vi "Papaleta.vi"() -> ()   [LabVIEW 2016]
doc: "Interfaz en Labview que emula la operación de un cajero automático basado en máquinas de estados por eventos, las cuales reducen el procesamiento de datos en el microprocesador.\nEsta cajero cuenta con las operaciones de Retiro de efectivo, Pago de tarjeta de crédito, Compra de tiempo Aire, Estado de cuenta, Donativos, Depósitos a otras cuentas y Salir, ademas de un inicio por contraseña por asteriscos."
uses:
  Control_1Enum.ctl
panel:
  out "unsigned 8bit integer":u8
  out "Tab Control":T1(tab)
  out "Anuncios":u8(ring)
  in  "Boton_Aceptar_Contrasena":bool
  in  "Contrasena":string
  in  "Salir":bool
  out "Adeudo_Tarjeta":dbl
  out "Credito_Disponible":dbl
  in  "Estado de cuenta":bool
  in  "Depositos a otras cuentas":bool
  in  "Donativos":bool
  in  "Comprar Tiempo Aire":bool
  in  "Pagar Tarjeta":bool
  in  "Retirar Efectivo":bool
  in  "Regresar_1":bool
  in  "Retirar_Efectivo":bool
  in  "Cantidad a Retirar":dbl min=0.0 max=10000.0
  out "Adeudo_Tarjeta 2":dbl
  out "Credito_Disponible 2":dbl
  in  "Regresar_2":bool
  in  "Monto_a_Pagar":dbl min=0.0 max=10000.0
  in  "Pago_Tarjeta_Crédito":bool
  out "Adeudo_Tarjeta 3":dbl
  out "Credito_Disponible 3":dbl
  in  "Regresar_3":bool
  out "Adeudo_Tarjeta 4":dbl
  out "Credito_Disponible 4":dbl
  in  "Recargar_100":bool
  in  "Recargar_200":bool
  in  "Recargar_300":bool
  in  "Recargar_500":bool
  in  "Regresar_4":bool
  out "Adeudo_Tarjeta 5":dbl
  out "Credito_Disponible 5":dbl
  in  "Donar 100":bool
  in  "Donar 200":bool
  in  "Donar 300":bool
  in  "Donar 500":bool
  in  "Fundacion a Donar":string(combo)="World Vision Mexico"
  in  "Regresar_5":bool
  in  "Boton_P":bool
  out "Cantidad":string
  in  "Persona a depositar":string(combo)="Adrian Barba"
  out "Adeudo_Tarjeta 6":dbl
  out "Credito_Disponible 6":dbl
  in  "Aceptar":bool
  in  "Borrar":bool
  in  "Boton_9":bool
  in  "Limpiar":bool
  in  "Boton_6":bool
  in  "Boton_0":bool
  in  "Boton_3":bool
  in  "Boton_8":bool
  in  "Boton_7":bool
  in  "Boton_5":bool
  in  "Boton_4":bool
  in  "Boton_2":bool
  in  "Boton_1":bool
  in  "Regresar_6":bool
  out "Transacciones":string
  in  "Inserte su tarjeta":bool
  out "Led_Parpadeante":bool
  # "BANCO NACIONAL DE UPIITA"
  # "INGRESE SU CLAVE"
  # "Contraseña"
  # "Operaciones a Realizar"
  # "Crédito Disponible"
  # "Adeudo de la Tarjeta"
  # "Retirar Crédito"
  # "Crédito Disponible"
  # "Adeudo de la Tarjeta"
  # "Realizar Pago de la Tarjeta"
  # "Crédito Disponible"
  # "Adeudo de la Tarjeta"
  # "Recargar Tiempo Aire"
  # "Crédito Disponible"
  # "Adeudo de la Tarjeta"
  # "Donaciones a la Caridad"
  # "Crédito Disponible"
  # "Adeudo de la Tarjeta"
  # "Adeudo de la Tarjeta"
  # "Crédito Disponible"
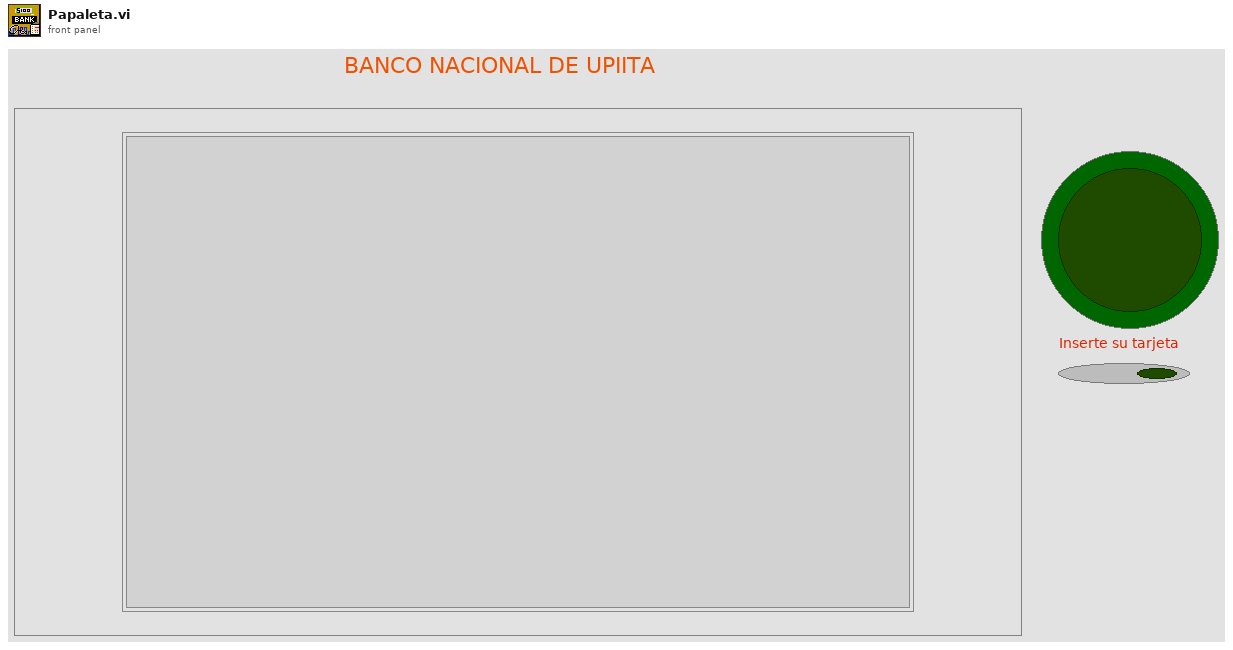
[diagram p1: front panel]
types:
  T1 = enum32{"Pant_Anuncios", "Pant_Contrasena", "Pant_Principal", "Pant_Retiro", "Pant_Pago", "Pant_Aire", "Pant_Donativos", "Pant_Depositos", "Pant_EdoCta"}
  T2 = typedef "Control_1Enum.ctl" = enum16{"Inicio", "Preguntar_Usuario", "Contrasena_valida", "Menu_Principal", "Menu_Retiro", "Menu_Pago", "Compra_TAire", "Donativos", "Depositos", "Estado_Cuenta"}
  T3 = cluster{"Credito Disponible":dbl, "Adeudo":dbl, "Primera Ejecucion":bool, "Transacciones":string, "Intentos":i8, "Pantalla":u8, "Cerrar Sesion":bool}
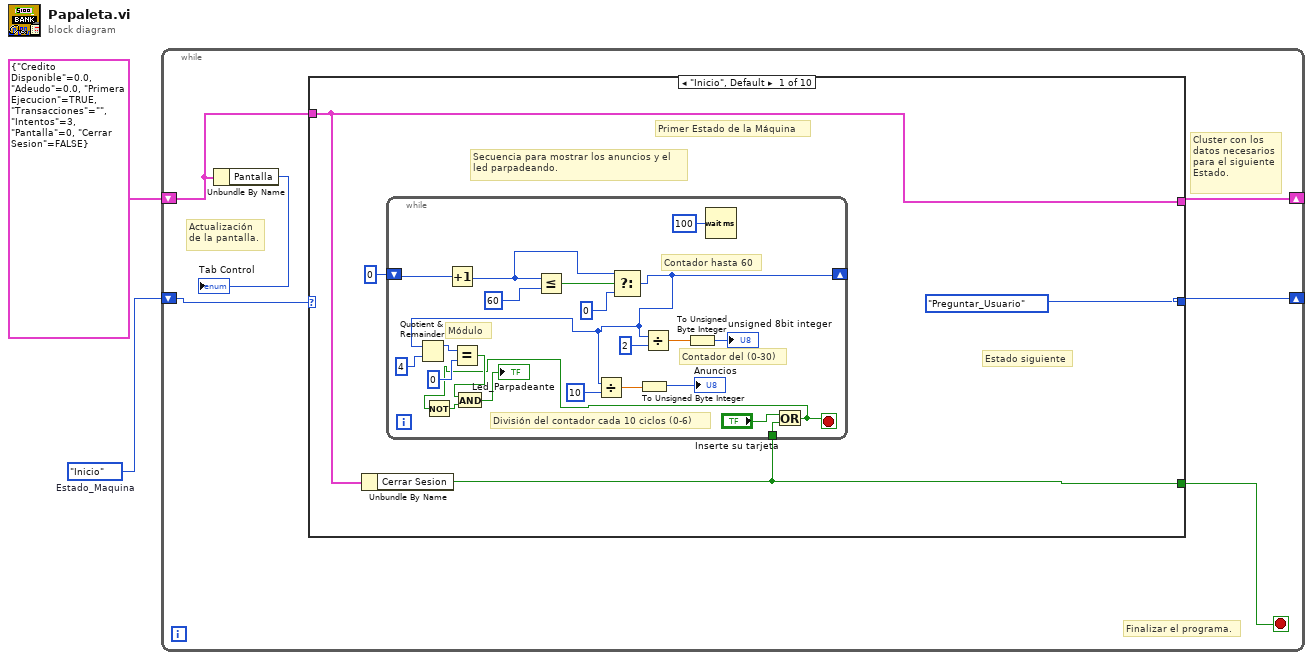
[diagram p0: block diagram]
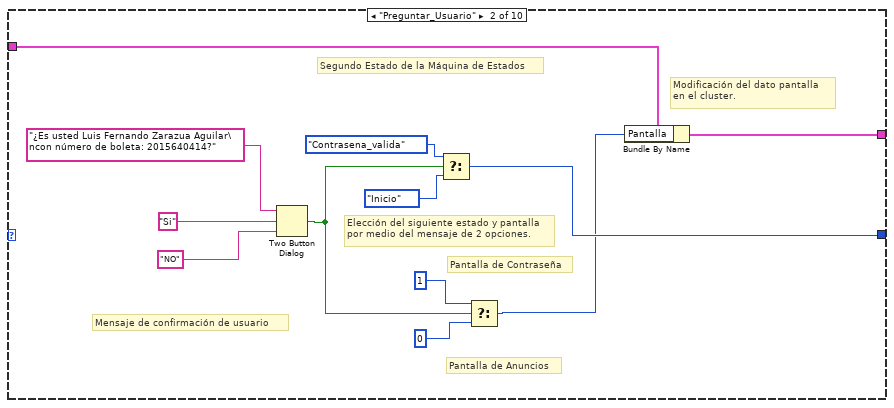
[diagram p2: hidden frame]
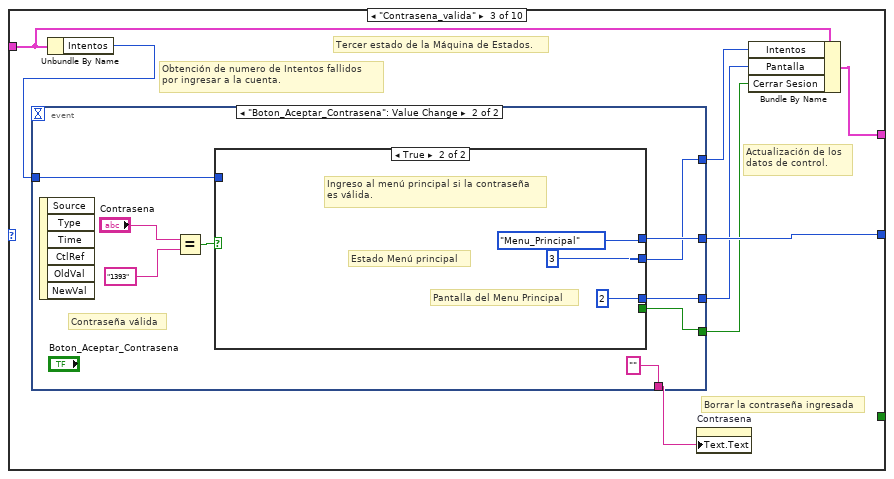
[diagram p3: hidden frame]
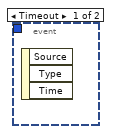
[diagram p4: hidden frame]
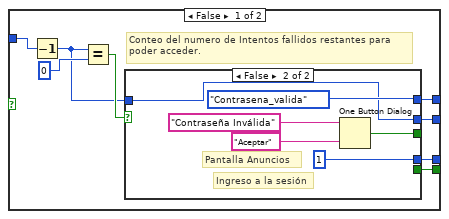
[diagram p5: hidden frame]
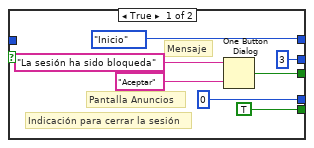
[diagram p6: hidden frame]
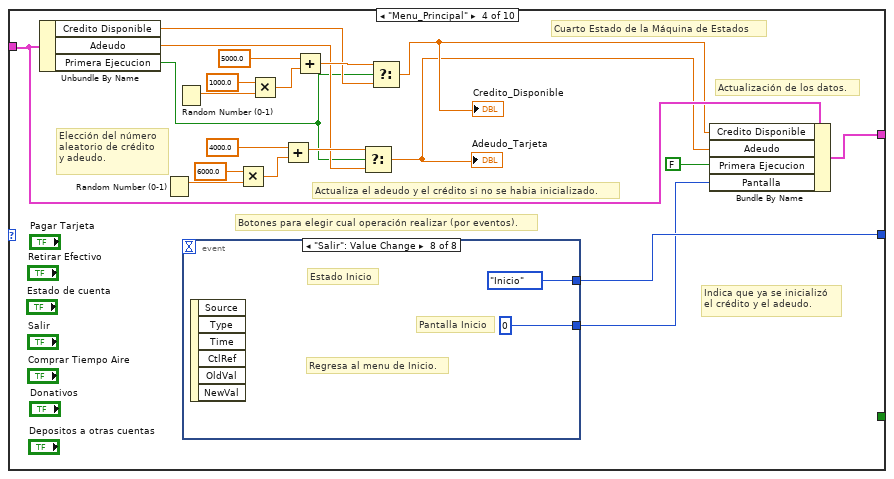
[diagram p7: hidden frame]
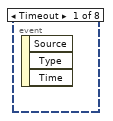
[diagram p8: hidden frame]
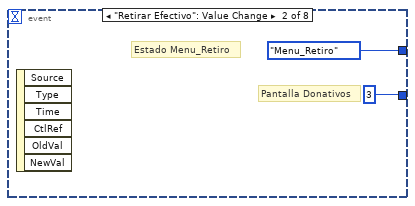
[diagram p9: hidden frame]
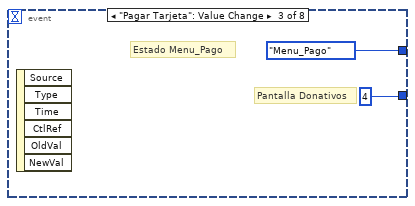
[diagram p10: hidden frame]
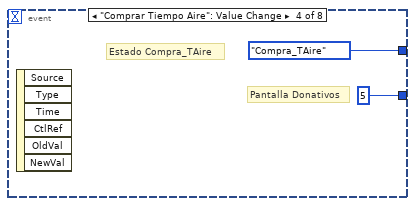
[diagram p11: hidden frame]
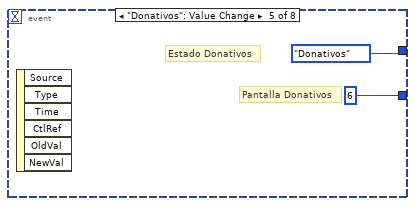
[diagram p12: hidden frame]
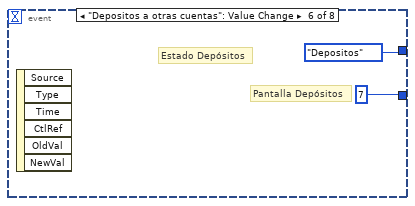
[diagram p13: hidden frame]
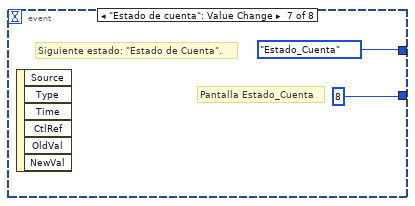
[diagram p14: hidden frame]
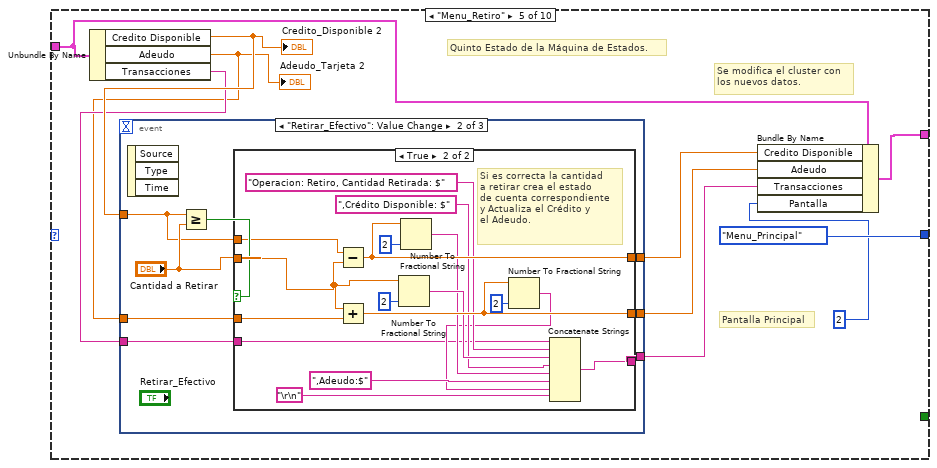
[diagram p15: hidden frame]
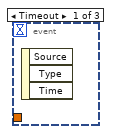
[diagram p16: hidden frame]
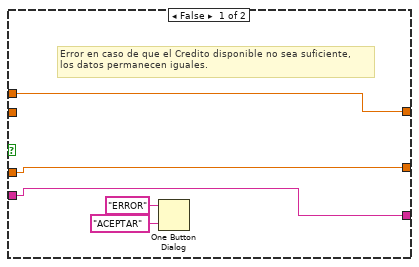
[diagram p17: hidden frame]
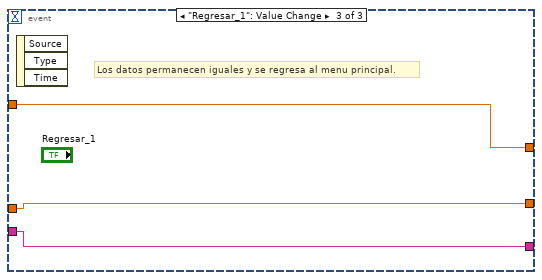
[diagram p18: hidden frame]
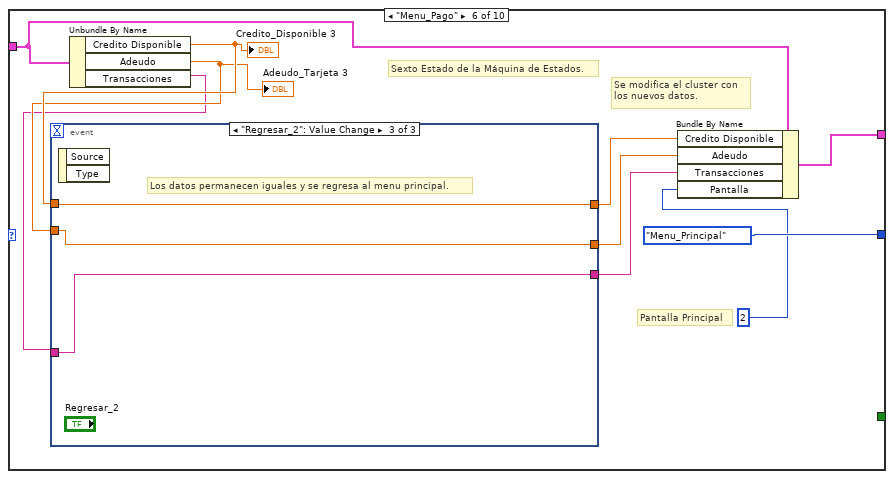
[diagram p19: hidden frame]
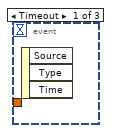
[diagram p20: hidden frame]
diagram:
  w2 = Control_1Enum."Inicio"  # Estado_Maquina
  n1 = while {
    shift-right: [w4] -> _
    shift-left: w2 -> [w3]
    shift-right: [w6] -> _
    shift-left: T3 {"Credito Disponible"=0.0, "Adeudo"=0.0, "Primera Ejecucion"=TRUE, "Transacciones"="", "Intentos"=3, "Pantalla"=0, "Cerrar Sesion"=FALSE} -> [w7]
    stop <- w5 stop-if-true
    # "Finalizar el programa."
    # "Cluster con los\ndatos necesarios\npara el siguiente\nEstado."
    # "Actualización \nde la pantalla."
    n2 = Unbundle By Name(w7) -> ("Pantalla"=→"Tab Control":u8)
    n3 = case shown="\"Inicio\", Default" w3 {
      tunnel: [Control_1Enum."Preguntar_Usuario" w40 w54 w97 Control_1Enum."Menu_Principal" Control_1Enum."Menu_Principal" Control_1Enum."Menu_Principal" Control_1Enum."Menu_Principal" w602 w774] -> w4
      tunnel: w7 -> [w10 w37 w51 w93 w123 w165 w211 w394 w584 w772]
      tunnel: [w10 w35 w49 w88 w122 w166 w210 w393 w583 w771] -> w6
      tunnel: [w9 _ _ _ _ _ _ _ _ _] -> w5
      frame "Inicio", Default {
        # "Secuencia para mostrar los anuncios y el\nled parpadeando."
        # "Estado siguiente"
        # "Primer Estado de la Máquina"
        n4 = Unbundle By Name(w10) -> ("Cerrar Sesion"=w9:bool)
        n5 = while {
          shift-right: [w22] -> _
          shift-left: i8 0 -> [w33]
          tunnel: w9 -> [w13]
          stop <- w15 stop-if-true
          # "Contador del (0-30)"
          # "Módulo"
          # "División del contador cada 10 ciclos (0-6)"
          # "Contador hasta 60"
          n6 = Increment(x=w33) -> (x+1=w30:i8)
          n7 = Less Or Equal?(x=w30, y=i8 60) -> (x <= y?=w31:bool)
          n8 = Select(t=w30, s=w31, f=i8 0) -> (s? t:f=w22:i8)
          n9 = Quotient & Remainder(x=w22, y=i8 4) -> (x-y*floor(x/y)=w20:i8)  [unwired: 1 out]
          n10 = Equal?(x=w20, y=i8 0) -> (x = y?=w17:bool)
          n11 = Divide(x=w22, y=i8 10) -> (x/y=w26:dbl)
          n12 = To Unsigned Byte Integer(number=w26) -> (unsigned 8bit integer=→"Anuncios":u8)
          n13 = Divide(x=w22, y=i8 2) -> (x/y=w24:dbl)
          n14 = To Unsigned Byte Integer(number=w24) -> (unsigned 8bit integer=→"unsigned 8bit integer":u8)
          n15 = Wait (ms)(milliseconds to wait=u32 100) -> ()  [unwired: 1 out]
          n16 = Or(x="Inserte su tarjeta", y=w13) -> (x .or. y?=w15:bool)
          n17 = Not(x=w15) -> (.not. x?=w16:bool)
          n18 = And(x=w17, y=w16) -> (x .and. y?=→"Led_Parpadeante":bool)
        }
      }
      frame "Preguntar_Usuario" {
        # "Modificación del dato pantalla\nen el cluster."
        # "Elección del siguiente estado y pantalla\npor medio del mensaje de 2 opciones."
        # "Mensaje de confirmación de usuario"
        # "Segundo Estado de la Máquina de Estados"
        # "Pantalla de Anuncios"
        # "Pantalla de Contraseña"
        n19 = Two Button Dialog(message="¿Es usted Luis Fernando Zarazua Aguilar\ncon número de boleta: 2015640414?", 1:"NO" ("F button name (\"Cancel\")"), 2:"Si" ("T button name (\"OK\")")) -> (T button?=w41:bool)
        n20 = Select(t=Control_1Enum."Contrasena_valida", s=w41, f=Control_1Enum."Inicio") -> (s? t:f=w40:T2)
        n21 = Select(t=u8 1, s=w41, f=0) -> (s? t:f=w36:i32)
        n22 = Bundle By Name(cluster=w37, "Pantalla"=w36) -> (w35:T3)
      }
      frame "Contrasena_valida" {
        # "Borrar la contraseña ingresada"
        # "Actualización de los\ndatos de control."
        # "Obtención de numero de Intentos fallidos\npor ingresar a la cuenta."
        # "Tercer estado de la Máquina de Estados."
        n23 = Unbundle By Name(w51) -> ("Intentos"=w52:i8)
        n24 = event shown="[1] \"Boton_Aceptar_Contrasena\": Value Change" {
          selector: _ -> [_ _]
          dyn-events: _ -> [_ _]
          timeout: _ -> [_ _]
          tunnel: [_ w60] -> w54
          tunnel: [_ w59] -> w48
          tunnel: [_ w58] -> w50
          tunnel: [_ "" ("Label.Text")] -> w53
          tunnel: [_ w56] -> w47
          tunnel: w52 -> [_ w55]
          event Timeout {
            n25 = event-data() -> ()  [unwired: 1 in, 3 out]
          }
          event "Boton_Aceptar_Contrasena": Value Change {
            # "Contraseña válida"
            n26 = event-data() -> ()  [unwired: 1 in, 6 out]
            n27 = Equal?(x="Contrasena", y="1393") -> (x = y?=w61:bool)
            n28 = case shown="True" w61 {
              tunnel: [w69 Control_1Enum."Menu_Principal"] -> w60
              tunnel: [w68 u8 2] -> w59
              tunnel: [w67 i8 3] -> w58
              tunnel: [w65 _] -> w56
              tunnel: w55 -> [w64 _]
              frame False {
                # "Conteo del numero de Intentos fallidos restantes para\npoder acceder."
                n29 = Decrement(x=w64) -> (x-1=w66:i8)
                n30 = Equal?(x=w66, y=i8 0) -> (x = y?=w70:bool)
                n31 = case shown="False" w70 {
                  tunnel: [Control_1Enum."Inicio" Control_1Enum."Contrasena_valida"] -> w69
                  tunnel: [u8 0 u8 1] -> w68
                  tunnel: [w74 w80] -> _
                  tunnel: [i8 3 w79] -> w67
                  tunnel: w66 -> [_ w79]
                  tunnel: [TRUE _] -> w65
                  frame True {
                    # "Mensaje"
                    # "Indicación para cerrar la sesión"
                    # "Pantalla Anuncios"
                    n32 = One Button Dialog(message="La sesión ha sido bloqueda", button name ("OK")="Aceptar") -> (true=w74:bool)
                  }
                  frame False {
                    # "Ingreso a la sesión"
                    # "Pantalla Anuncios"
                    n33 = One Button Dialog(message="Contraseña Inválida", button name ("OK")="Aceptar") -> (true=w80:bool)
                  }
                }
              }
              frame True {
                # "Estado Menú principal"
                # "Ingreso al menú principal si la contraseña\nes válida."
                # "Pantalla del Menu Principal"
              }
            }
          }
        }
        n34 = property on="Contrasena" class="Str"("Text.Text"=w53) -> ()  [unwired: 2 in, 2 out]
        n35 = Bundle By Name(cluster=w51, "Intentos"=w50, "Pantalla"=w48, "Cerrar Sesion"=w47) -> (w49:T3)
      }
      frame "Menu_Principal" {
        # "Actualización de los datos."
        # "Indica que ya se inicializó \nel crédito y el adeudo."
        # "Botones para elegir cual operación realizar (por eventos)."
        # "Actualiza el adeudo y el crédito si no se habia inicializado."
        # "Elección del número\naleatorio de crédito\ny adeudo."
        # "Cuarto Estado de la Máquina de Estados"
        n36 = Unbundle By Name(w93) -> ("Credito Disponible"=w96:dbl, "Adeudo"=w95:dbl, "Primera Ejecucion"=w94:bool)
        n37 = Random Number (0-1)() -> (number: 0 to 1=w103:dbl)
        n38 = Random Number (0-1)() -> (number: 0 to 1=w107:dbl)
        n39 = event shown="[7] \"Salir\": Value Change" {
          selector: _ -> [_ _ _ _ _ _ _ _]
          dyn-events: _ -> [_ _ _ _ _ _ _ _]
          timeout: _ -> [_ _ _ _ _ _ _ _]
          tunnel: [_ Control_1Enum."Menu_Retiro" Control_1Enum."Menu_Pago" Control_1Enum."Compra_TAire" Control_1Enum."Donativos" Control_1Enum."Depositos" Control_1Enum."Estado_Cuenta" Control_1Enum."Inicio"] -> w97
          tunnel: [_ u8 3 u8 4 u8 5 u8 6 u8 7 u8 8 u8 0] -> w89
          event Timeout {
            n40 = event-data() -> ()  [unwired: 1 in, 3 out]
          }
          event "Retirar Efectivo": Value Change {
            # "Estado Menu_Retiro"
            # "Pantalla Donativos"
            n41 = event-data() -> ()  [unwired: 1 in, 6 out]
          }
          event "Pagar Tarjeta": Value Change {
            # "Estado Menu_Pago"
            # "Pantalla Donativos"
            n42 = event-data() -> ()  [unwired: 1 in, 6 out]
          }
          event "Comprar Tiempo Aire": Value Change {
            # "Estado Compra_TAire"
            # "Pantalla Donativos"
            n43 = event-data() -> ()  [unwired: 1 in, 6 out]
          }
          event "Donativos": Value Change {
            # "Estado Donativos"
            # "Pantalla Donativos"
            n44 = event-data() -> ()  [unwired: 1 in, 6 out]
          }
          event "Depositos a otras cuentas": Value Change {
            # "Estado Depósitos"
            # "Pantalla Depósitos"
            n45 = event-data() -> ()  [unwired: 1 in, 6 out]
          }
          event "Estado de cuenta": Value Change {
            # "Siguiente estado: \"Estado de Cuenta\"."
            # "Pantalla Estado_Cuenta"
            n46 = event-data() -> ()  [unwired: 1 in, 6 out]
          }
          event "Salir": Value Change {
            # "Regresa al menu de Inicio."
            # "Estado Inicio"
            # "Pantalla Inicio"
            n47 = event-data() -> ()  [unwired: 1 in, 6 out]
          }
        }
        n48 = Multiply(x=6000.0, y=w103) -> (x*y=w100:dbl)
        n49 = Multiply(x=1000.0, y=w107) -> (x*y=w104:dbl)
        n50 = Add(x=4000.0, y=w100) -> (x+y=w98:dbl)
        n51 = Add(x=5000.0, y=w104) -> (x+y=w99:dbl)
        n52 = Select(t=w98, s=w94, f=w95) -> (s? t:f=w91:dbl)
        "Adeudo_Tarjeta" <- w91
        n53 = Select(t=w99, s=w94, f=w96) -> (s? t:f=w92:dbl)
        "Credito_Disponible" <- w92
        n54 = Bundle By Name(cluster=w93, "Credito Disponible"=w92, "Adeudo"=w91, "Primera Ejecucion"=FALSE, "Pantalla"=w89) -> (w88:T3)
      }
      frame "Menu_Retiro" {
        # "Se modifica el cluster con\nlos nuevos datos."
        # "Quinto Estado de la Máquina de Estados."
        # "Pantalla Principal"
        n55 = Unbundle By Name(w123) -> ("Credito Disponible"=w126:dbl, "Adeudo"=w124:dbl, "Transacciones"=w125:string)
        "Credito_Disponible 2" <- w126
        "Adeudo_Tarjeta 2" <- w124
        n56 = event shown="[1] \"Retirar_Efectivo\": Value Change" {
          selector: _ -> [_ _ _]
          dyn-events: _ -> [_ _ _]
          timeout: _ -> [_ _ _]
          tunnel: [_ w137 w164] -> w129
          tunnel: [_ w136 w163] -> w127
          tunnel: [_ w135 w162] -> w128
          tunnel: w126 -> [_ w132 w164]
          tunnel: w125 -> [_ w134 w162]
          tunnel: w124 -> [_ w133 w163]
          event Timeout {
            n57 = event-data() -> ()  [unwired: 1 in, 3 out]
          }
          event "Retirar_Efectivo": Value Change {
            n58 = event-data() -> ()  [unwired: 1 in, 3 out]
            n59 = Greater Or Equal?(x=w132, y="Cantidad a Retirar") -> (x >= y?=w138:bool)
            n60 = case shown="True" w138 {
              tunnel: "Cantidad a Retirar" -> [_ w155]
              tunnel: [w141 w159] -> w136
              tunnel: [w142 w158] -> w137
              tunnel: [w140 w161] -> w135
              tunnel: w134 -> [w140 w147]
              tunnel: w133 -> [w141 w146]
              tunnel: w132 -> [w142 w145]
              frame False {
                # "Error en caso de que el Credito disponible no sea suficiente,\nlos datos permanecen iguales."
                n61 = One Button Dialog(message="ERROR", button name ("OK")="ACEPTAR") -> ()  [unwired: 1 out]
              }
              frame True {
                # "Si es correcta la cantidad\na retirar crea el estado\nde cuenta correspondiente\ny Actualiza el Crédito y\nel Adeudo."
                n62 = Subtract(x=w145, y=w155) -> (x-y=w158:dbl)
                n63 = Add(x=w155, y=w146) -> (x+y=w159:dbl)
                n64 = Number To Fractional String(number=w155, precision (6)=i16 2 ("width (-)")) -> (F-format string=w153:string)  [unwired: 2 in]
                n65 = Number To Fractional String(number=w158, precision (6)=i16 2 ("width (-)")) -> (F-format string=w151:string)  [unwired: 2 in]
                n66 = Number To Fractional String(number=w159, precision (6)=i16 2 ("width (-)")) -> (F-format string=w149:string)  [unwired: 2 in]
                n67 = Concatenate Strings(w147, "Operacion: Retiro, Cantidad Retirada: $" ("string"), w153, ",Crédito Disponible: $" ("string"), w151, ",Adeudo:$" ("string"), w149, "\r\n") -> (w161:string)
              }
            }
          }
          event "Regresar_1": Value Change {
            # "Los datos permanecen iguales y se regresa al menu principal."
            n68 = event-data() -> ()  [unwired: 1 in, 3 out]
          }
        }
        n69 = Bundle By Name(cluster=w123, "Credito Disponible"=w129, "Adeudo"=w127, "Transacciones"=w128, "Pantalla"=u8 2) -> (w122:T3)
      }
      frame "Menu_Pago" {
        # "Se modifica el cluster con\nlos nuevos datos."
        # "Sexto Estado de la Máquina de Estados."
        # "Pantalla Principal"
        n70 = Unbundle By Name(w165) -> ("Credito Disponible"=w173:dbl, "Adeudo"=w172:dbl, "Transacciones"=w171:string)
        "Adeudo_Tarjeta 3" <- w172
        "Credito_Disponible 3" <- w173
        n71 = event shown="[2] \"Regresar_2\": Value Change" {
          selector: _ -> [_ _ _]
          dyn-events: _ -> [_ _ _]
          timeout: _ -> [_ _ _]
          tunnel: [_ w180 w209] -> w167
          tunnel: [_ w179 w208] -> w168
          tunnel: [_ w178 w207] -> w169
          tunnel: w173 -> [_ w176 w209]
          tunnel: w172 -> [_ w175 w208]
          tunnel: w171 -> [_ w177 w207]
          event Timeout {
            n72 = event-data() -> ()  [unwired: 1 in, 3 out]
          }
          event "Pago_Tarjeta_Crédito": Value Change {
            # "Realiza la comparación del Crédito disponible y del adeudo"
            n73 = event-data() -> ()  [unwired: 1 in, 2 out]
            n74 = Less Or Equal?(x="Monto_a_Pagar", y=w176) -> (x <= y?=w184:bool)
            n75 = Less Or Equal?(x="Monto_a_Pagar", y=w175) -> (x <= y?=w183:bool)
            n76 = And(x=w184, y=w183) -> (x .and. y?=w182:bool)
            n77 = case shown="False" w182 {
              tunnel: "Monto_a_Pagar" -> [_ w197]
              tunnel: [w186 w195] -> w179
              tunnel: [w187 w196] -> w180
              tunnel: [w185 w194] -> w178
              tunnel: w177 -> [w185 w192]
              tunnel: w176 -> [w187 w191]
              tunnel: w175 -> [w186 w190]
              frame False {
                # "Si es falso se manda un mensaje de error y los datos\ndatos quedan igual."
                n78 = One Button Dialog(message="Error al Pagar", button name ("OK")="Aceptar") -> ()  [unwired: 1 out]
              }
              frame True {
                # "Si es correcto se actualizan los datos."
                n79 = Add(x=w191, y=w197) -> (x+y=w196:dbl)
                n80 = Subtract(x=w190, y=w197) -> (x-y=w195:dbl)
                n81 = Number To Fractional String(number=w197, precision (6)=i16 2 ("width (-)")) -> (F-format string=w203:string)  [unwired: 2 in]
                n82 = Number To Fractional String(number=w196, precision (6)=i16 2 ("width (-)")) -> (F-format string=w201:string)  [unwired: 2 in]
                n83 = Number To Fractional String(number=w195, precision (6)=i16 2 ("width (-)")) -> (F-format string=w199:string)  [unwired: 2 in]
                n84 = Concatenate Strings(w192, "Operacion: Pago de Tarjeta, Cantidad Ingresada: $" ("string"), w203, ",Crédito Disponible: $" ("string"), w201, ",Adeudo:$" ("string"), w199, "\r\n") -> (w194:string)
              }
            }
          }
          event "Regresar_2": Value Change {
            # "Los datos permanecen iguales y se regresa al menu principal."
            n85 = event-data() -> ()  [unwired: 1 in, 2 out]
          }
        }
        n86 = Bundle By Name(cluster=w165, "Credito Disponible"=w167, "Adeudo"=w168, "Transacciones"=w169, "Pantalla"=u8 2) -> (w166:T3)
      }
      frame "Compra_TAire" {
        # "Se modifica el cluster con\nlos nuevos datos."
        # "Se obtienen los datos guardados\nnecesarios para la operación."
        # "Séptimo Estado de la Máquina de Estados."
        # "Pantalla Principal"
        n87 = Unbundle By Name(w211) -> ("Credito Disponible"=w217:dbl, "Adeudo"=w216:dbl, "Transacciones"=w218:string)
        "Credito_Disponible 4" <- w217
        "Adeudo_Tarjeta 4" <- w216
        n88 = event shown="[4] \"Recargar_500\": Value Change" {
          selector: _ -> [_ _ _ _ _ _]
          dyn-events: _ -> [_ _ _ _ _ _]
          timeout: _ -> [_ _ _ _ _ _]
          tunnel: [_ w238 w278 w318 w358 w388] -> w212
          tunnel: [_ w237 w277 w317 w357 w386] -> w213
          tunnel: "\r\n" -> [_ w231 w271 w311 w351 _]
          tunnel: ", Deuda: $" -> [_ w232 w272 w312 w352 _]
          tunnel: ", Crédito Disponible: $" -> [_ w233 w273 w313 w353 _]
          tunnel: ", Deuda Anterior: $" -> [_ w234 w274 w314 w354 _]
          tunnel: ", Crédito Anterior: $" -> [_ w235 w275 w315 w355 _]
          tunnel: "Operación: Recarga de Tiempo Aire, Cantidad Recargada: $" -> [_ w236 w276 w316 w356 _]
          tunnel: [_ w230 w270 w310 w350 w387] -> w214
          tunnel: w218 -> [_ w229 w269 w309 w349 w387]
          tunnel: w216 -> [_ w228 w268 w308 w348 w386]
          tunnel: w217 -> [_ w227 w267 w307 w347 w388]
          event Timeout {
            n89 = event-data() -> ()  [unwired: 1 in, 3 out]
          }
          event "Recargar_100": Value Change {
            w239 = 100.0 ("y")
            n90 = event-data() -> ()  [unwired: 1 in, 1 out]
            n91 = Greater Or Equal?(x=w227, y=w239) -> (x >= y?=w226:bool)
            n92 = case shown="True" w226 {
              tunnel: [w241 w263] -> w237
              tunnel: [w242 w260] -> w238
              tunnel: w239 -> [_ w264]
              tunnel: w236 -> [_ w257]
              tunnel: w235 -> [_ w255]
              tunnel: w234 -> [_ w253]
              tunnel: w233 -> [_ w250]
              tunnel: w232 -> [_ w249]
              tunnel: w231 -> [_ w247]
              tunnel: [w240 w246] -> w230
              tunnel: w229 -> [w240 w245]
              tunnel: w228 -> [w241 w244]
              tunnel: w227 -> [w242 w243]
              frame False {
                # "Los datos permanecen iguales\n y se regresa al menu principal."
              }
              frame True {
                # "Se actualizan\nlos datos si\nes correcto."
                n93 = Subtract(x=w243, y=w264) -> (x-y=w260:dbl)
                n94 = Add(x=w264, y=w244) -> (x+y=w263:dbl)
                n95 = Number To Fractional String(number=w244, precision (6)=i16 2) -> (F-format string=w252:string)  [unwired: 2 in]
                n96 = Number To Fractional String(number=w243, precision (6)=i16 2) -> (F-format string=w254:string)  [unwired: 2 in]
                n97 = Number To Fractional String(number=w264, precision (6)=i16 2) -> (F-format string=w256:string)  [unwired: 2 in]
                n98 = Number To Fractional String(number=w260, precision (6)=i16 2) -> (F-format string=w251:string)  [unwired: 2 in]
                n99 = Number To Fractional String(number=w263, precision (6)=i16 2) -> (F-format string=w248:string)  [unwired: 2 in]
                n100 = Concatenate Strings(w245, w257, w256, w255, w254, w253, w252, w250, w251, w249, w248, w247) -> (w246:string)
              }
            }
          }
          event "Recargar_200": Value Change {
            w279 = 200.0 ("y")
            n101 = event-data() -> ()  [unwired: 1 in, 1 out]
            n102 = Greater Or Equal?(x=w267, y=w279) -> (x >= y?=w266:bool)
            n103 = case shown="False" w266 {
              tunnel: [w281 w303] -> w277
              tunnel: [w282 w300] -> w278
              tunnel: w279 -> [_ w304]
              tunnel: w276 -> [_ w297]
              tunnel: w275 -> [_ w295]
              tunnel: w274 -> [_ w293]
              tunnel: w273 -> [_ w290]
              tunnel: w272 -> [_ w289]
              tunnel: w271 -> [_ w287]
              tunnel: [w280 w286] -> w270
              tunnel: w269 -> [w280 w285]
              tunnel: w268 -> [w281 w284]
              tunnel: w267 -> [w282 w283]
              frame False {
                # "Los datos permanecen iguales\n y se regresa al menu principal."
              }
              frame True {
                # "Se actualizan\nlos datos si\nes correcto."
                n104 = Subtract(x=w283, y=w304) -> (x-y=w300:dbl)
                n105 = Add(x=w304, y=w284) -> (x+y=w303:dbl)
                n106 = Number To Fractional String(number=w284, precision (6)=i16 2) -> (F-format string=w292:string)  [unwired: 2 in]
                n107 = Number To Fractional String(number=w283, precision (6)=i16 2) -> (F-format string=w294:string)  [unwired: 2 in]
                n108 = Number To Fractional String(number=w304, precision (6)=i16 2) -> (F-format string=w296:string)  [unwired: 2 in]
                n109 = Number To Fractional String(number=w300, precision (6)=i16 2) -> (F-format string=w291:string)  [unwired: 2 in]
                n110 = Number To Fractional String(number=w303, precision (6)=i16 2) -> (F-format string=w288:string)  [unwired: 2 in]
                n111 = Concatenate Strings(w285, w297, w296, w295, w294, w293, w292, w290, w291, w289, w288, w287) -> (w286:string)
              }
            }
          }
          event "Recargar_300": Value Change {
            w319 = 300.0 ("y")
            n112 = event-data() -> ()  [unwired: 1 in, 1 out]
            n113 = Greater Or Equal?(x=w307, y=w319) -> (x >= y?=w306:bool)
            n114 = case shown="False" w306 {
              tunnel: [w321 w343] -> w317
              tunnel: [w322 w340] -> w318
              tunnel: w319 -> [_ w344]
              tunnel: w316 -> [_ w337]
              tunnel: w315 -> [_ w335]
              tunnel: w314 -> [_ w333]
              tunnel: w313 -> [_ w330]
              tunnel: w312 -> [_ w329]
              tunnel: w311 -> [_ w327]
              tunnel: [w320 w326] -> w310
              tunnel: w309 -> [w320 w325]
              tunnel: w308 -> [w321 w324]
              tunnel: w307 -> [w322 w323]
              frame False {
                # "Los datos permanecen iguales\n y se regresa al menu principal."
              }
              frame True {
                # "Se actualizan\nlos datos si\nes correcto."
                n115 = Subtract(x=w323, y=w344) -> (x-y=w340:dbl)
                n116 = Add(x=w344, y=w324) -> (x+y=w343:dbl)
                n117 = Number To Fractional String(number=w324, precision (6)=i16 2) -> (F-format string=w332:string)  [unwired: 2 in]
                n118 = Number To Fractional String(number=w323, precision (6)=i16 2) -> (F-format string=w334:string)  [unwired: 2 in]
                n119 = Number To Fractional String(number=w344, precision (6)=i16 2) -> (F-format string=w336:string)  [unwired: 2 in]
                n120 = Number To Fractional String(number=w340, precision (6)=i16 2) -> (F-format string=w331:string)  [unwired: 2 in]
                n121 = Number To Fractional String(number=w343, precision (6)=i16 2) -> (F-format string=w328:string)  [unwired: 2 in]
                n122 = Concatenate Strings(w325, w337, w336, w335, w334, w333, w332, w330, w331, w329, w328, w327) -> (w326:string)
              }
            }
          }
          event "Recargar_500": Value Change {
            w359 = 500.0 ("y")
            n123 = event-data() -> ()  [unwired: 1 in, 1 out]
            n124 = Greater Or Equal?(x=w347, y=w359) -> (x >= y?=w346:bool)
            n125 = case shown="False" w346 {
              tunnel: [w361 w383] -> w357
              tunnel: [w362 w380] -> w358
              tunnel: w359 -> [_ w384]
              tunnel: w356 -> [_ w377]
              tunnel: w355 -> [_ w375]
              tunnel: w354 -> [_ w373]
              tunnel: w353 -> [_ w370]
              tunnel: w352 -> [_ w369]
              tunnel: w351 -> [_ w367]
              tunnel: [w360 w366] -> w350
              tunnel: w349 -> [w360 w365]
              tunnel: w348 -> [w361 w364]
              tunnel: w347 -> [w362 w363]
              frame False {
                # "Los datos permanecen iguales\n y se regresa al menu principal."
              }
              frame True {
                # "Se actualizan\nlos datos si\nes correcto."
                n126 = Subtract(x=w363, y=w384) -> (x-y=w380:dbl)
                n127 = Add(x=w384, y=w364) -> (x+y=w383:dbl)
                n128 = Number To Fractional String(number=w364, precision (6)=i16 2) -> (F-format string=w372:string)  [unwired: 2 in]
                n129 = Number To Fractional String(number=w363, precision (6)=i16 2) -> (F-format string=w374:string)  [unwired: 2 in]
                n130 = Number To Fractional String(number=w384, precision (6)=i16 2) -> (F-format string=w376:string)  [unwired: 2 in]
                n131 = Number To Fractional String(number=w380, precision (6)=i16 2) -> (F-format string=w371:string)  [unwired: 2 in]
                n132 = Number To Fractional String(number=w383, precision (6)=i16 2) -> (F-format string=w368:string)  [unwired: 2 in]
                n133 = Concatenate Strings(w365, w377, w376, w375, w374, w373, w372, w370, w371, w369, w368, w367) -> (w366:string)
              }
            }
          }
          event "Regresar_3": Value Change {
            # "Los datos permanecen iguales y se regresa al menu principal."
            n134 = event-data() -> ()  [unwired: 1 in, 1 out]
          }
        }
        n135 = Bundle By Name(cluster=w211, "Credito Disponible"=w212, "Adeudo"=w213, "Transacciones"=w214, "Pantalla"=u8 2) -> (w210:T3)
      }
      frame "Donativos" {
        # "Se obtienen los datos guardados\nnecesarios para la operación."
        # "Se modifica el cluster con\nlos nuevos datos."
        # "Noveno Estado de la Máquina de Estados."
        # "Pantalla Principal"
        n136 = Unbundle By Name(w394) -> ("Credito Disponible"=w391:dbl, "Adeudo"=w392:dbl, "Transacciones"=w399:string)
        "Credito_Disponible 5" <- w391
        "Adeudo_Tarjeta 5" <- w392
        n137 = event shown="[5] \"Regresar_4\": Value Change" {
          selector: _ -> [_ _ _ _ _ _]
          dyn-events: _ -> [_ _ _ _ _ _]
          timeout: _ -> [_ _ _ _ _ _]
          tunnel: "\r\n" -> [_ w421 w464 w507 w550 _]
          tunnel: ", Deuda: $" -> [_ w420 w463 w506 w549 _]
          tunnel: ", Crédito Disponible: $" -> [_ w419 w462 w505 w548 _]
          tunnel: ", Deuda Anterior: $" -> [_ w418 w461 w504 w547 _]
          tunnel: ", Crédito Anterior: $" -> [_ w417 w460 w503 w546 _]
          tunnel: [_ w416 w459 w502 w545 w579] -> w398
          tunnel: [_ w415 w458 w501 w544 w580] -> w396
          tunnel: [_ w414 w457 w500 w543 w578] -> w397
          tunnel: w399 -> [_ w413 w456 w499 w542 w580]
          tunnel: w392 -> [_ w412 w455 w498 w541 w578]
          tunnel: w391 -> [_ w411 w454 w497 w540 w579]
          tunnel: ", Cantidad Donada: $" -> [_ w408 w451 w494 w537 _]
          tunnel: "Operación: Donación a " -> [_ w406 w449 w492 w535 _]
          event Timeout {
            n138 = event-data() -> ()  [unwired: 1 in, 3 out]
          }
          event "Donar 100": Value Change {
            w422 = 100.0 ("y")
            n139 = event-data() -> ()  [unwired: 1 in, 1 out]
            n140 = property on="Fundacion a Donar" class="CmbBox"() -> ("Text.Text"=w407:string)  [unwired: 2 in, 2 out]
            n141 = Concatenate Strings(w406, w407, w408) -> (w409:string)
            n142 = Greater Or Equal?(x=w411, y=w422) -> (x >= y?=w410:bool)
            n143 = case shown="False" w410 {
              tunnel: [w424 w446] -> w414
              tunnel: [w425 w443] -> w416
              tunnel: w422 -> [_ w447]
              tunnel: w409 -> [_ w440]
              tunnel: w417 -> [_ w438]
              tunnel: w418 -> [_ w436]
              tunnel: w419 -> [_ w433]
              tunnel: w420 -> [_ w432]
              tunnel: w421 -> [_ w430]
              tunnel: [w423 w429] -> w415
              tunnel: w413 -> [w423 w428]
              tunnel: w411 -> [w425 w427]
              tunnel: w412 -> [w424 w426]
              frame False {
                # "Los datos permanecen iguales\n y se regresa al menu principal."
              }
              frame True {
                # "Se actualizan\nlos datos si\nes correcto."
                n144 = Subtract(x=w427, y=w447) -> (x-y=w443:dbl)
                n145 = Add(x=w447, y=w426) -> (x+y=w446:dbl)
                n146 = Number To Fractional String(number=w426, precision (6)=i16 2) -> (F-format string=w435:string)  [unwired: 2 in]
                n147 = Number To Fractional String(number=w427, precision (6)=i16 2) -> (F-format string=w437:string)  [unwired: 2 in]
                n148 = Number To Fractional String(number=w447, precision (6)=i16 2) -> (F-format string=w439:string)  [unwired: 2 in]
                n149 = Number To Fractional String(number=w443, precision (6)=i16 2) -> (F-format string=w434:string)  [unwired: 2 in]
                n150 = Number To Fractional String(number=w446, precision (6)=i16 2) -> (F-format string=w431:string)  [unwired: 2 in]
                n151 = Concatenate Strings(w428, w440, w439, w438, w437, w436, w435, w433, w434, w432, w431, w430) -> (w429:string)
              }
            }
          }
          event "Donar 200": Value Change {
            w465 = 200.0 ("y")
            n152 = event-data() -> ()  [unwired: 1 in, 1 out]
            n153 = property on="Fundacion a Donar" class="CmbBox"() -> ("Text.Text"=w450:string)  [unwired: 2 in, 2 out]
            n154 = Concatenate Strings(w449, w450, w451) -> (w452:string)
            n155 = Greater Or Equal?(x=w454, y=w465) -> (x >= y?=w453:bool)
            n156 = case shown="False" w453 {
              tunnel: [w467 w489] -> w457
              tunnel: [w468 w486] -> w459
              tunnel: w465 -> [_ w490]
              tunnel: w452 -> [_ w483]
              tunnel: w460 -> [_ w481]
              tunnel: w461 -> [_ w479]
              tunnel: w462 -> [_ w476]
              tunnel: w463 -> [_ w475]
              tunnel: w464 -> [_ w473]
              tunnel: [w466 w472] -> w458
              tunnel: w456 -> [w466 w471]
              tunnel: w454 -> [w468 w470]
              tunnel: w455 -> [w467 w469]
              frame False {
                # "Los datos permanecen iguales\n y se regresa al menu principal."
              }
              frame True {
                # "Se actualizan\nlos datos si\nes correcto."
                n157 = Subtract(x=w470, y=w490) -> (x-y=w486:dbl)
                n158 = Add(x=w490, y=w469) -> (x+y=w489:dbl)
                n159 = Number To Fractional String(number=w469, precision (6)=i16 2) -> (F-format string=w478:string)  [unwired: 2 in]
                n160 = Number To Fractional String(number=w470, precision (6)=i16 2) -> (F-format string=w480:string)  [unwired: 2 in]
                n161 = Number To Fractional String(number=w490, precision (6)=i16 2) -> (F-format string=w482:string)  [unwired: 2 in]
                n162 = Number To Fractional String(number=w486, precision (6)=i16 2) -> (F-format string=w477:string)  [unwired: 2 in]
                n163 = Number To Fractional String(number=w489, precision (6)=i16 2) -> (F-format string=w474:string)  [unwired: 2 in]
                n164 = Concatenate Strings(w471, w483, w482, w481, w480, w479, w478, w476, w477, w475, w474, w473) -> (w472:string)
              }
            }
          }
          event "Donar 300": Value Change {
            w508 = 300.0 ("y")
            n165 = event-data() -> ()  [unwired: 1 in, 1 out]
            n166 = property on="Fundacion a Donar" class="CmbBox"() -> ("Text.Text"=w493:string)  [unwired: 2 in, 2 out]
            n167 = Concatenate Strings(w492, w493, w494) -> (w495:string)
            n168 = Greater Or Equal?(x=w497, y=w508) -> (x >= y?=w496:bool)
            n169 = case shown="False" w496 {
              tunnel: [w510 w532] -> w500
              tunnel: [w511 w529] -> w502
              tunnel: w508 -> [_ w533]
              tunnel: w495 -> [_ w526]
              tunnel: w503 -> [_ w524]
              tunnel: w504 -> [_ w522]
              tunnel: w505 -> [_ w519]
              tunnel: w506 -> [_ w518]
              tunnel: w507 -> [_ w516]
              tunnel: [w509 w515] -> w501
              tunnel: w499 -> [w509 w514]
              tunnel: w497 -> [w511 w513]
              tunnel: w498 -> [w510 w512]
              frame False {
                # "Los datos permanecen iguales\n y se regresa al menu principal."
              }
              frame True {
                # "Se actualizan\nlos datos si\nes correcto."
                n170 = Subtract(x=w513, y=w533) -> (x-y=w529:dbl)
                n171 = Add(x=w533, y=w512) -> (x+y=w532:dbl)
                n172 = Number To Fractional String(number=w512, precision (6)=i16 2) -> (F-format string=w521:string)  [unwired: 2 in]
                n173 = Number To Fractional String(number=w513, precision (6)=i16 2) -> (F-format string=w523:string)  [unwired: 2 in]
                n174 = Number To Fractional String(number=w533, precision (6)=i16 2) -> (F-format string=w525:string)  [unwired: 2 in]
                n175 = Number To Fractional String(number=w529, precision (6)=i16 2) -> (F-format string=w520:string)  [unwired: 2 in]
                n176 = Number To Fractional String(number=w532, precision (6)=i16 2) -> (F-format string=w517:string)  [unwired: 2 in]
                n177 = Concatenate Strings(w514, w526, w525, w524, w523, w522, w521, w519, w520, w518, w517, w516) -> (w515:string)
              }
            }
          }
          event "Donar 500": Value Change {
            w551 = 500.0 ("y")
            n178 = event-data() -> ()  [unwired: 1 in, 1 out]
            n179 = property on="Fundacion a Donar" class="CmbBox"() -> ("Text.Text"=w536:string)  [unwired: 2 in, 2 out]
            n180 = Concatenate Strings(w535, w536, w537) -> (w538:string)
            n181 = Greater Or Equal?(x=w540, y=w551) -> (x >= y?=w539:bool)
            n182 = case shown="False" w539 {
              tunnel: [w553 w575] -> w543
              tunnel: [w554 w572] -> w545
              tunnel: w551 -> [_ w576]
              tunnel: w538 -> [_ w569]
              tunnel: w546 -> [_ w567]
              tunnel: w547 -> [_ w565]
              tunnel: w548 -> [_ w562]
              tunnel: w549 -> [_ w561]
              tunnel: w550 -> [_ w559]
              tunnel: [w552 w558] -> w544
              tunnel: w542 -> [w552 w557]
              tunnel: w540 -> [w554 w556]
              tunnel: w541 -> [w553 w555]
              frame False {
                # "Los datos permanecen iguales\n y se regresa al menu principal."
              }
              frame True {
                # "Se actualizan\nlos datos si\nes correcto."
                n183 = Subtract(x=w556, y=w576) -> (x-y=w572:dbl)
                n184 = Add(x=w576, y=w555) -> (x+y=w575:dbl)
                n185 = Number To Fractional String(number=w555, precision (6)=i16 2) -> (F-format string=w564:string)  [unwired: 2 in]
                n186 = Number To Fractional String(number=w556, precision (6)=i16 2) -> (F-format string=w566:string)  [unwired: 2 in]
                n187 = Number To Fractional String(number=w576, precision (6)=i16 2) -> (F-format string=w568:string)  [unwired: 2 in]
                n188 = Number To Fractional String(number=w572, precision (6)=i16 2) -> (F-format string=w563:string)  [unwired: 2 in]
                n189 = Number To Fractional String(number=w575, precision (6)=i16 2) -> (F-format string=w560:string)  [unwired: 2 in]
                n190 = Concatenate Strings(w557, w569, w568, w567, w566, w565, w564, w562, w563, w561, w560, w559) -> (w558:string)
              }
            }
          }
          event "Regresar_4": Value Change {
            # "Los datos permanecen iguales y se regresa al menu principal."
            n191 = event-data() -> ()  [unwired: 1 in, 2 out]
          }
        }
        n192 = Bundle By Name(cluster=w394, "Credito Disponible"=w398, "Adeudo"=w397, "Transacciones"=w396, "Pantalla"=u8 2) -> (w393:T3)
      }
      frame "Depositos" {
        w592 = -1.0 ("default (0 DBL)")
        # "Se obtienen los datos guardados\nnecesarios para la operación."
        # "Convierte a numero\nel caracter ingresado."
        # "Obtiene la persona a quien se le depositará."
        # "Se modifica el cluster con\nlos nuevos datos."
        # "Décimo Estado de la Máquina de Estados."
        n193 = Unbundle By Name(w584) -> ("Credito Disponible"=w590:dbl, "Adeudo"=w589:dbl, "Transacciones"=w591:string)
        "Credito_Disponible 6" <- w590
        "Adeudo_Tarjeta 6" <- w589
        n194 = property on="Cantidad" class="Str"() -> ("Text.Text"=w594:string)  [unwired: 2 in, 2 out]
        n195 = Fract/Exp String To Number(use system decimal point (T)=TRUE, string=w594, default (0 dbl)=w592) -> (number=w593:dbl)  [unwired: 1 in, 1 out]
        n196 = event shown="[14] \"Regresar_5\": Value Change" {
          selector: _ -> [_ _ _ _ _ _ _ _ _ _ _ _ _ _ _]
          dyn-events: _ -> [_ _ _ _ _ _ _ _ _ _ _ _ _ _ _]
          timeout: _ -> [_ _ _ _ _ _ _ _ _ _ _ _ _ _ _]
          tunnel: [w608 w616 w624 w632 w640 w648 w656 w664 w672 w680 w688 w696 "" w717 w767] -> w595
          tunnel: [Control_1Enum."Depositos" Control_1Enum."Depositos" Control_1Enum."Depositos" Control_1Enum."Depositos" Control_1Enum."Depositos" Control_1Enum."Depositos" Control_1Enum."Depositos" Control_1Enum."Depositos" Control_1Enum."Depositos" Control_1Enum."Depositos" Control_1Enum."Depositos" Control_1Enum."Depositos" Control_1Enum."Depositos" w719 Control_1Enum."Menu_Principal"] -> w602
          tunnel: [u8 7 u8 7 u8 7 u8 7 u8 7 u8 7 u8 7 u8 7 u8 7 u8 7 u8 7 u8 7 u8 7 w718 u8 2] -> w588
          tunnel: ", Crédito Anterior: $" -> [_ _ _ _ _ _ _ _ _ _ _ _ _ w729 _]
          tunnel: ", Deuda Anterior: $" -> [_ _ _ _ _ _ _ _ _ _ _ _ _ w728 _]
          tunnel: ", Crédito Disponible: $" -> [_ _ _ _ _ _ _ _ _ _ _ _ _ w727 _]
          tunnel: ", Deuda: $" -> [_ _ _ _ _ _ _ _ _ _ _ _ _ w726 _]
          tunnel: "\r\n" -> [_ _ _ _ _ _ _ _ _ _ _ _ _ w725 _]
          tunnel: w593 -> [_ _ _ _ _ _ _ _ _ _ _ _ _ w720 _]
          tunnel: w592 -> [_ _ _ _ _ _ _ _ _ _ _ _ _ w724 _]
          tunnel: [w606 w611 w619 w627 w635 w643 w651 w659 w667 w675 w683 w691 w701 w716 w764] -> w587
          tunnel: [w605 w613 w621 w629 w637 w645 w653 w661 w669 w677 w685 w693 w703 w715 w766] -> w585
          tunnel: [w604 w612 w620 w628 w636 w644 w652 w660 w668 w676 w684 w692 w702 w714 w765] -> w586
          tunnel: w591 -> [w606 w611 w619 w627 w635 w643 w651 w659 w667 w675 w683 w691 w701 w711 w764]
          tunnel: w590 -> [w605 w613 w621 w629 w637 w645 w653 w661 w669 w677 w685 w693 w703 w712 w766]
          tunnel: w589 -> [w604 w612 w620 w628 w636 w644 w652 w660 w668 w676 w684 w692 w702 w713 w765]
          tunnel: ", Cantidad Donada: $" -> [_ _ _ _ _ _ _ _ _ _ _ _ _ w710 _]
          tunnel: "Operación: Depósito a " -> [_ _ _ _ _ _ _ _ _ _ _ _ _ w709 _]
          event "Boton_0": Value Change {
            # "Ingresa el numero \"0\" al display."
            # "Pantalla Depósitos"
            n197 = event-data() -> ()  [unwired: 1 in, 2 out]
            n198 = property on="Cantidad" class="Str"() -> ("Text.Text"=w610:string)  [unwired: 2 in, 2 out]
            n199 = Concatenate Strings(w610, "0") -> (w608:string)
          }
          event "Boton_1": Value Change {
            # "Ingresa el numero \"1\" al display."
            # "Pantalla Depósitos"
            n200 = event-data() -> ()  [unwired: 1 in, 2 out]
            n201 = property on="Cantidad" class="Str"() -> ("Text.Text"=w618:string)  [unwired: 2 in, 2 out]
            n202 = Concatenate Strings(w618, "1") -> (w616:string)
          }
          event "Boton_2": Value Change {
            # "Ingresa el numero \"2\" al display."
            # "Pantalla Depósitos"
            n203 = event-data() -> ()  [unwired: 1 in, 2 out]
            n204 = property on="Cantidad" class="Str"() -> ("Text.Text"=w626:string)  [unwired: 2 in, 2 out]
            n205 = Concatenate Strings(w626, "2") -> (w624:string)
          }
          event "Boton_3": Value Change {
            # "Ingresa el numero \"3\" al display."
            # "Pantalla Depósitos"
            n206 = event-data() -> ()  [unwired: 1 in, 3 out]
            n207 = property on="Cantidad" class="Str"() -> ("Text.Text"=w634:string)  [unwired: 2 in, 2 out]
            n208 = Concatenate Strings(w634, "3") -> (w632:string)
          }
          event "Boton_4": Value Change {
            # "Ingresa el numero \"4\" al display."
            # "Pantalla Depósitos"
            n209 = event-data() -> ()  [unwired: 1 in, 3 out]
            n210 = property on="Cantidad" class="Str"() -> ("Text.Text"=w642:string)  [unwired: 2 in, 2 out]
            n211 = Concatenate Strings(w642, "4") -> (w640:string)
          }
          event "Boton_5": Value Change {
            # "Ingresa el numero \"5\" al display."
            # "Pantalla Depósitos"
            n212 = event-data() -> ()  [unwired: 1 in, 3 out]
            n213 = property on="Cantidad" class="Str"() -> ("Text.Text"=w650:string)  [unwired: 2 in, 2 out]
            n214 = Concatenate Strings(w650, "5") -> (w648:string)
          }
          event "Boton_6": Value Change {
            # "Ingresa el numero \"6\" al display."
            # "Pantalla Depósitos"
            n215 = event-data() -> ()  [unwired: 1 in, 3 out]
            n216 = property on="Cantidad" class="Str"() -> ("Text.Text"=w658:string)  [unwired: 2 in, 2 out]
            n217 = Concatenate Strings(w658, "6") -> (w656:string)
          }
          event "Boton_7": Value Change {
            # "Ingresa el numero \"7\" al display."
            # "Pantalla Depósitos"
            n218 = event-data() -> ()  [unwired: 1 in, 3 out]
            n219 = property on="Cantidad" class="Str"() -> ("Text.Text"=w666:string)  [unwired: 2 in, 2 out]
            n220 = Concatenate Strings(w666, "7") -> (w664:string)
          }
          event "Boton_8": Value Change {
            # "Ingresa el numero \"8\" al display."
            # "Pantalla Depósitos"
            n221 = event-data() -> ()  [unwired: 1 in, 3 out]
            n222 = property on="Cantidad" class="Str"() -> ("Text.Text"=w674:string)  [unwired: 2 in, 2 out]
            n223 = Concatenate Strings(w674, "8") -> (w672:string)
          }
          event "Boton_9": Value Change {
            # "Ingresa el numero \"9\" al display."
            # "Pantalla Depósitos"
            n224 = event-data() -> ()  [unwired: 1 in, 3 out]
            n225 = property on="Cantidad" class="Str"() -> ("Text.Text"=w682:string)  [unwired: 2 in, 2 out]
            n226 = Concatenate Strings(w682, "9") -> (w680:string)
          }
          event "Boton_P": Value Change {
            # "Ingresa el punto decimal al display."
            # "Pantalla Depósitos"
            n227 = event-data() -> ()  [unwired: 1 in, 2 out]
            n228 = property on="Cantidad" class="Str"() -> ("Text.Text"=w690:string)  [unwired: 2 in, 2 out]
            n229 = Concatenate Strings(w690, ".") -> (w688:string)
          }
          event "Borrar": Value Change {
            # "Este boton borra un caracter anterior,\nverificando si todavia hay alguno."
            # "Pantalla Depósitos"
            n230 = event-data() -> ()  [unwired: 1 in, 2 out]
            n231 = property on="Cantidad" class="Str"() -> ("Text.Text"=w697:string)  [unwired: 2 in, 2 out]
            n232 = String Length(string=w697) -> (length=w694:i32)
            n233 = Decrement(x=w694) -> (x-1=w695:i32)
            n234 = String Subset(string=w697, offset (0)=0, length (rest)=w695) -> (substring=w696:string)
          }
          event "Limpiar": Value Change {
            # "Este boton limpia la pantalla."
            # "Pantalla Depósitos"
            n235 = event-data() -> ()  [unwired: 1 in, 2 out]
          }
          event "Aceptar": Value Change {
            n236 = event-data() -> ()  [unwired: 1 in, 1 out]
            n237 = Greater Or Equal?(x=w712, y=w720) -> (x >= y?=w723:bool)
            n238 = Greater?(x=w720, y=w724) -> (0:w722:bool)
            n239 = property on="Persona a depositar" class="CmbBox"() -> ("Text.Text"=w708:string)  [unwired: 2 in, 2 out]
            n240 = Concatenate Strings(w709, w708, w710) -> (w707:string)
            n241 = And(x=w723, y=w722) -> (x .and. y?=w721:bool)
            n242 = case shown="True" w721 {
              tunnel: [w730 w762] -> w714
              tunnel: [w732 w759] -> w715
              tunnel: w707 -> [w731 w756]
              tunnel: w729 -> [_ w754]
              tunnel: w728 -> [_ w752]
              tunnel: w727 -> [_ w749]
              tunnel: w726 -> [_ w748]
              tunnel: w725 -> [_ w746]
              tunnel: [w731 w745] -> w716
              tunnel: w720 -> [_ w740]
              tunnel: [Control_1Enum."Depositos" Control_1Enum."Menu_Principal"] -> w719
              tunnel: [u8 7 u8 2] -> w718
              tunnel: [w735 ""] -> w717
              tunnel: w713 -> [w730 w738]
              tunnel: w712 -> [w732 w741]
              tunnel: w711 -> [_ w739]
              frame False {
                # "En caso contrario se\nse indica un error y \nse permanece en el\nmismo estado."
                # "Pantalla Depósitos"
                n243 = property on="Cantidad" class="Str"() -> ("Text.Text"=w735:string)  [unwired: 2 in, 2 out]
                n244 = One Button Dialog(message="Datos Inválidos", button name ("OK")="Aceptar") -> ()  [unwired: 1 out]
              }
              frame True {
                # "Se actualizan\nlos datos si\nes correcto."
                # "P. Principal"
                n245 = Subtract(x=w741, y=w740) -> (x-y=w759:dbl)
                n246 = Add(x=w740, y=w738) -> (x+y=w762:dbl)
                n247 = Number To Fractional String(number=w738, precision (6)=i16 2) -> (F-format string=w751:string)  [unwired: 2 in]
                n248 = Number To Fractional String(number=w741, precision (6)=i16 2) -> (F-format string=w753:string)  [unwired: 2 in]
                n249 = Number To Fractional String(number=w740, precision (6)=i16 2) -> (F-format string=w755:string)  [unwired: 2 in]
                n250 = Number To Fractional String(number=w759, precision (6)=i16 2) -> (F-format string=w750:string)  [unwired: 2 in]
                n251 = Number To Fractional String(number=w762, precision (6)=i16 2) -> (F-format string=w747:string)  [unwired: 2 in]
                n252 = Concatenate Strings(w739, w756, w755, w754, w753, w752, w751, w749, w750, w748, w747, w746) -> (w745:string)
              }
            }
          }
          event "Regresar_5": Value Change {
            # "Los datos permanecen iguales y se regresa al menu principal."
            # "Pantalla Principal"
            n253 = event-data() -> ()  [unwired: 1 in, 2 out]
            n254 = property on="Cantidad" class="Str"() -> ("Text.Text"=w767:string)  [unwired: 2 in, 2 out]
          }
        }
        "Cantidad" <- w595
        n255 = Bundle By Name(cluster=w584, "Credito Disponible"=w585, "Adeudo"=w586, "Transacciones"=w587, "Pantalla"=w588) -> (w583:T3)
      }
      frame "Estado_Cuenta" {
        # "Se obtienen los datos guardados\nnecesarios para la operación."
        # "Onceavo Estado de la Máquina de Estados."
        # "Se muestran las transacciones realizadas."
        n256 = Unbundle By Name(w772) -> ("Transacciones"=→"Transacciones":string)
        n257 = event shown="[1] \"Regresar_6\": Value Change" {
          selector: _ -> [_ _]
          dyn-events: _ -> [_ _]
          timeout: _ -> [_ _]
          tunnel: [_ Control_1Enum."Menu_Principal"] -> w774
          tunnel: [_ u8 2] -> w770
          event Timeout {
            n258 = event-data() -> ()  [unwired: 1 in, 3 out]
          }
          event "Regresar_6": Value Change {
            # "Los datos permanecen iguales y se regresa al menu principal."
            # "Pantalla Principal"
            n259 = event-data() -> ()  [unwired: 1 in, 6 out]
          }
        }
        n260 = Bundle By Name(cluster=w772, "Pantalla"=w770) -> (w771:T3)
      }
    }
  }
